vi "Neocera Get Parameters.vi"(8 "error in (no error)":errorcluster, 10 "Control Panel Data":T1={"Record heater"=FALSE, "Record RAW"=FALSE, "Set point"=0.0, "Heater range"=0.0, "Approach"=enum."Instant", "Ramp rate, K/min"=0.0, "Record Channels"=[], "Settling time "=60.0, "Settling range"=0.1, "P"=0.0, "I"=0.0, "D"=0.0, "Temperature Control"=FALSE}, 11 "VISA resource name":refnum<visa-resource-name>) -> (0 "error out":errorcluster, 2 "Control Panel Data Out":T1={"Record heater"=FALSE, "Record RAW"=FALSE, "Set point"=0.0, "Heater range"=0.0, "Approach"=enum."Instant", "Ramp rate, K/min"=0.0, "Record Channels"=[], "Settling time "=60.0, "Settling range"=0.1, "P"=0.0, "I"=0.0, "D"=0.0, "Temperature Control"=FALSE}, 3 "VISA Resource Name Out":refnum<visa-resource-name>)   [LabVIEW 2015]
uses:
  Mag Lab Measure/Hardware/Temperarture Controller/T controller parameters.ctl
  Neocera Set Point Aproach.ctl
  GPIB/VISA  Send Receive.vi
panel:
  out "data string 2":string
  out "data string out":string
  # "Temperature Monitor"
  # "Temperature Monitor"
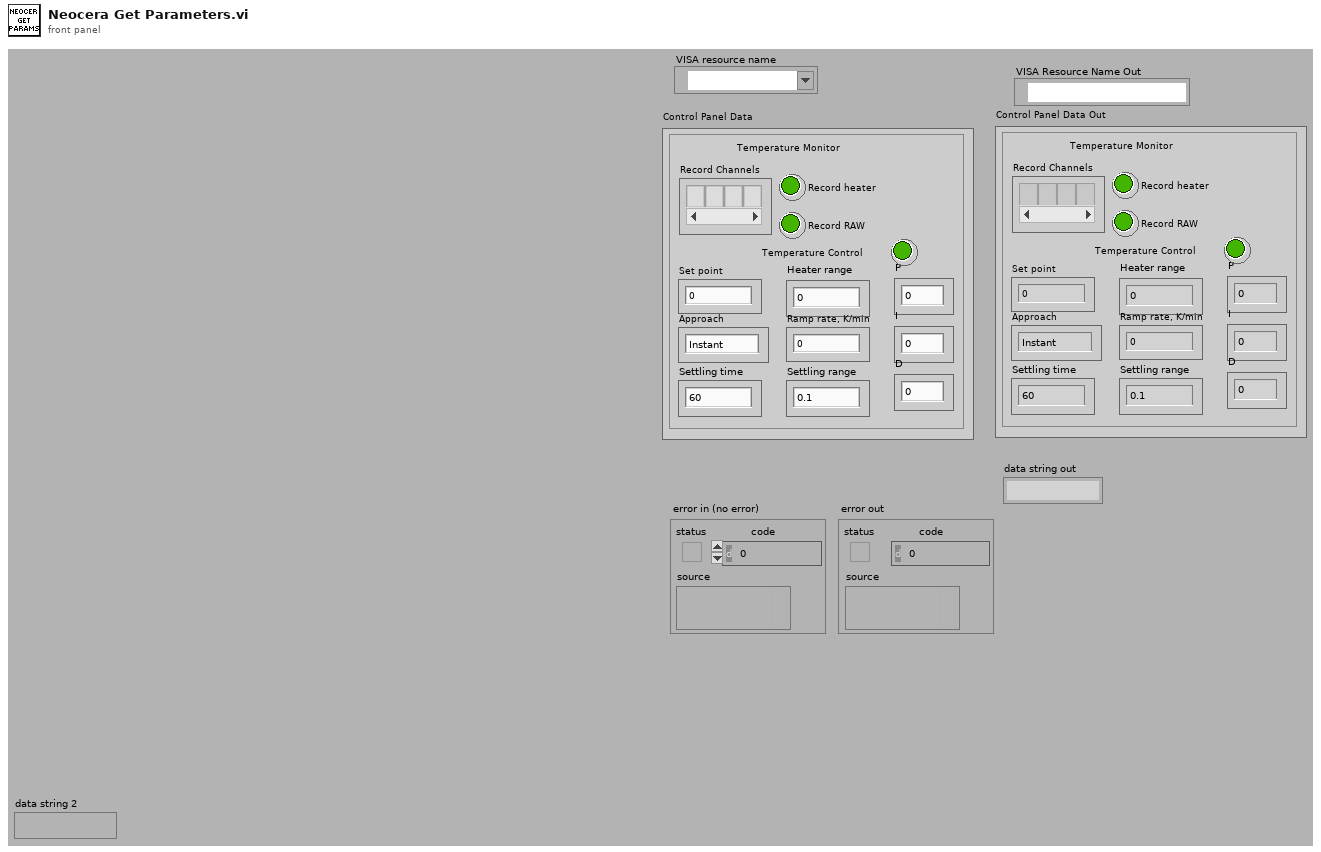
[diagram p1: front panel]
types:
  T1 = typedef "T controller parameters.ctl" = cluster{"Record heater":bool, "Record RAW":bool, "Set point":dbl, "Heater range":dbl, "Approach":T2, "Ramp rate, K/min":dbl, "Record Channels":string[], "Settling time ":dbl, "Settling range":dbl, "P":dbl, "I":dbl, "D":dbl, "Temperature Control":bool}
  T2 = typedef "Neocera Set Point Aproach.ctl" = enum16{"Instant", "Ramp"}
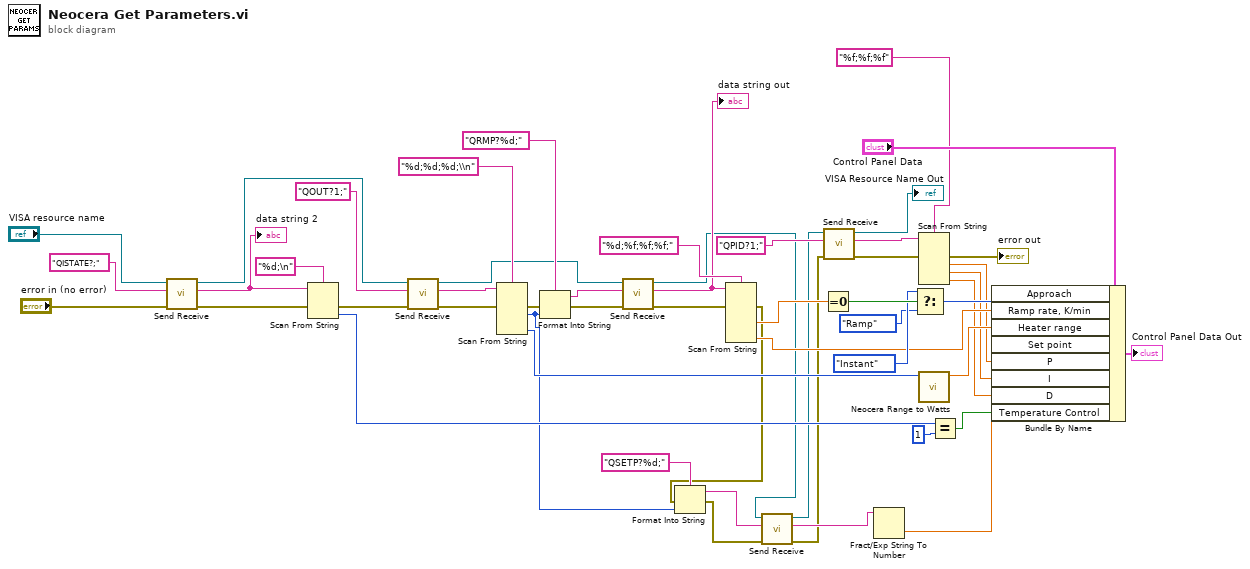
[diagram p0: block diagram]
diagram:
  n1 = call-poly "Send Receive.vi"("error in (no error)"="error in (no error)", "data string in"="QISTATE?;" ("data string"), "VISA Resource Name"="VISA resource name") -> ("error out"=w48:errorcluster, "data string out"=w44:string, "VISA Resource Name Out"=w33:refnum<visa-resource-name>)  [unwired: 6 in]
  "data string 2" <- w44
  n2 = Scan From String(format string="%d;\n", input string=w44, error in=w48) -> (error out=w38:errorcluster, output 1=w46:i32)  [unwired: 2 in, 2 out]
  n3 = call-poly "Send Receive.vi"("error in (no error)"=w38, "data string in"="QOUT?1;", "VISA Resource Name"=w33) -> ("error out"=w37:errorcluster, "data string out"=w35:string, "VISA Resource Name Out"=w34:refnum<visa-resource-name>)  [unwired: 6 in]
  n4 = Scan From String(format string="%d;%d;%d;\\n", input string=w35, error in=w37) -> (error out=w36:errorcluster, output 1=w9:i32, output 3=w16:i32)  [unwired: 5 in, 2 out]
  n5 = Format Into String(format string="QRMP?%d;", error in=w36, w9) -> (resulting string=w41:string, error out=w42:errorcluster)  [unwired: 1 in]
  n6 = call-poly "Send Receive.vi"("error in (no error)"=w42, "data string in"=w41, "VISA Resource Name"=w34) -> ("error out"=w40:errorcluster, "data string out"=w12:string, "VISA Resource Name Out"=w6:refnum<visa-resource-name>)  [unwired: 6 in]
  "data string out" <- w12
  n7 = Scan From String(format string="%d;%f;%f;%f;", input string=w12, error in=w40) -> (error out=w8:errorcluster, output 2=w31:dbl, output 4=w20:dbl)  [unwired: 7 in, 2 out]
  n8 = Format Into String(format string="QSETP?%d;", error in=w8, w9) -> (resulting string=w4:string, error out=w7:errorcluster)  [unwired: 1 in]
  n9 = call-poly "Send Receive.vi"("error in (no error)"=w7, "data string in"=w4, "VISA Resource Name"=w6) -> ("error out"=w1:errorcluster, "data string out"=w3:string, "VISA Resource Name Out"=w5:refnum<visa-resource-name>)  [unwired: 6 in]
  n10 = Equal To 0?(x=w31) -> (x = 0?=w30:bool)
  n11 = call-poly "Send Receive.vi"("error in (no error)"=w1, "data string in"="QPID?1;" ("write buffer"), "VISA Resource Name"=w5) -> ("error out"=w24:errorcluster, "data string out"=w25:string, "VISA Resource Name Out"=→"VISA Resource Name Out":refnum<visa-resource-name>)  [unwired: 6 in]
  n12 = Fract/Exp String To Number(string=w3) -> (number=w2:dbl)  [unwired: 3 in, 1 out]
  n13 = Select(t=Neocera_Set_Point_Aproach."Instant" ("Approach"), s=w30, f=Neocera_Set_Point_Aproach."Ramp" ("Approach")) -> (s? t:f=w21:T2)
  n14 = Scan From String(format string="%f;%f;%f", input string=w25, error in=w24) -> (error out=→"error out":errorcluster, output 1=w19:dbl, output 2=w18:dbl, output 3=w17:dbl)  [unwired: 4 in, 2 out]
  n15 = call "Neocera Range to Watts.vi"("Integer range"=w16) -> ("Watts"=w50:dbl)  [unwired: 9 in, 1 out]
  n16 = Equal?(x=w46, y=1) -> (x = y?=w15:bool)
  n17 = Bundle By Name(cluster="Control Panel Data", "Approach"=w21, "Ramp rate, K/min"=w20, "Heater range"=w50, "Set point"=w2, "P"=w19, "I"=w18, "D"=w17, "Temperature Control"=w15) -> (→"Control Panel Data Out":T1)
